vi "RFH-convert-r140.vi"(5 "Destination Folder":path, 7 "Folder Path":path, 11 "Xi":dbl[](array[numeric])) -> (0 "error out":errorcluster)   [LabVIEW 2020, in "RFH-Reflection_File_Handler.lvlib"]
uses:
  RFH-Reflection_File_Handler.lvlib
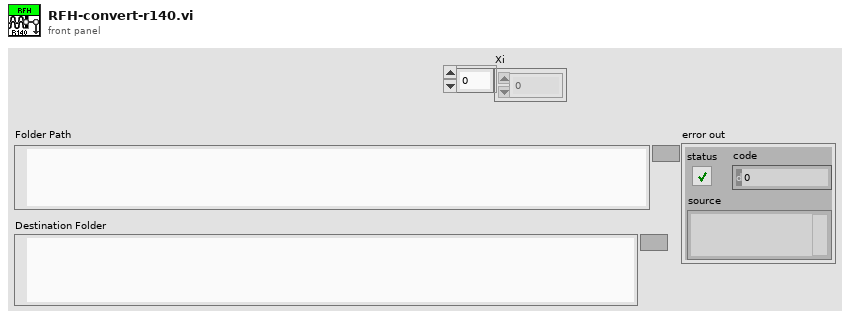
[diagram p1: front panel]
types:
  T1 = typedef "RFH-Reflection_File_Handler.lvlib/RFH-common_data_format.ctl" = cluster{"Frequency":dbl[], "Reflection'":dbl[], "Reflection''":dbl[], "Permativity'":dbl[], "Permativity''":dbl[]}
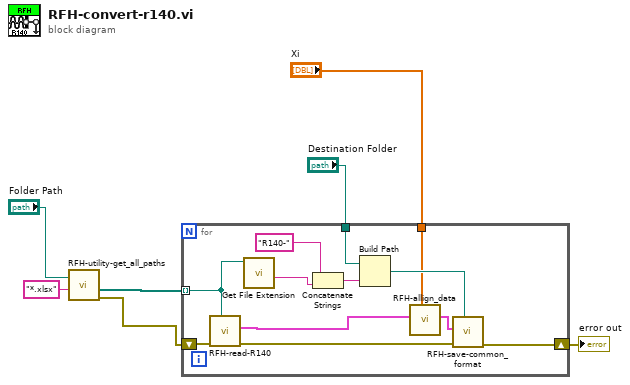
[diagram p0: block diagram]
diagram:
  n1 = call "RFH-utility-get_all_paths.vi"("Folder Path"="Folder Path", "pattern"="*.xlsx") -> ("error out"=w4:errorcluster, "All Files in Dir"=w7:path[])  [unwired: 6 in, 2 out]
  n2 = for {
    tunnel: w7 -> [w19] mode=indexing
    tunnel: "Destination Folder" -> [w16]
    shift-right: [w12] -> w3
    shift-left: w4 -> [w11]
    tunnel: "Xi" -> [w8]
    n3 = call "RFH-read-R140.vi"("file path (dialog if empty)"=w19, "error in (no error)"=w11) -> ("error out"=w13:errorcluster, "Common Format"=w10:T1)  [unwired: 7 in, 1 out]
    n4 = call <vilib>:"Get File Extension.vi"("file"=w19) -> ("filename without extension"=w18:string)  [unwired: 6 in, 4 out]
    n5 = Concatenate Strings("R140-" ("string"), w18) -> (w17:string)
    n6 = Build Path(base path=w16, name or relative path=w17) -> (appended path=w14:path)
    n7 = call "RFH-allign_data.vi"("Xi"=w8, "Common Format"=w10) -> ("Common Format alligned"=w9:T1)  [unwired: 9 in]
    n8 = call "RFH-save-common_format.vi"("file path (use dialog)"=w14, "error in (no error)"=w13, "Common Format"=w9) -> ("error out"=w12:errorcluster)  [unwired: 8 in]
  }
  "error out" <- w3
